vi "Get Proto Value from Enum Value.vi"(8 "error in (no error)":errorcluster, 9 "enum name":string, 10 "value in LV":u32, 11 "gRPC ID in":T1) -> (0 "error out":errorcluster, 2 "value in proto":i32, 3 "gRPC ID out":T1)   [LabVIEW 2019, in "grpc-lvsupport.lvlib"]
uses:
  grpc-lvsupport.lvlib
  grpcId.ctl
  <vilib>/Utility/file.llb/Application Directory.vi
  <vilib>/Utility/error.llb/Error Cluster From Error Code.vi
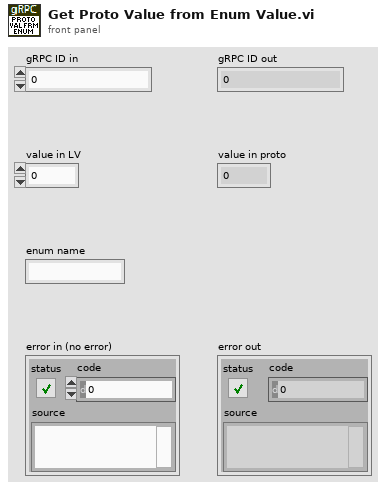
[diagram p1: front panel]
types:
  T1 = typedef "grpc-lvsupport.lvlib/grpcId.ctl" = u64
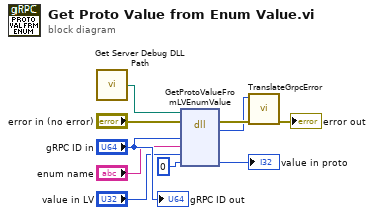
[diagram p0: block diagram]
diagram:
  n1 = call "Get Server Debug DLL Path.vi"() -> ("DLL Path"=w9:path)
  n2 = dll-call lib="?" fn="GetProtoValueFromLVEnumValue"(path in=w9, error in="error in (no error)", "gRPC ID in"="gRPC ID in", "enum name"="enum name", "value in LV"="value in LV", "value in proto"=0) -> (error out=w7:errorcluster, "error code"=w6:i32, "value in proto"=→"value in proto":i32)  [unwired: 4 in, 1 out]
  n3 = call "TranslateGrpcError.vi"("error in"=w7, "Error Code"=w6) -> ("error out"=→"error out":errorcluster)  [unwired: 9 in]
  "gRPC ID out" <- "gRPC ID in"
